vi "I(V)_MFLI_PK_v4.0_measure X_JA.vi"() -> ()   [LabVIEW 2016]
uses:
  <instrlib>/Zurich Instruments LabOne/Public/Data/ziTypeDemodSampleSingle.ctl
  <instrlib>/Zurich Instruments LabOne/Public/Configure/ziSetValueDouble.vi
  <instrlib>/Zurich Instruments LabOne/Public/Configure/ziGetValueDemodSampleEx.vi
  <instrlib>/Zurich Instruments LabOne/Zurich Instruments LabOne.lvlib
panel:
  in  "MFLI Average":i32=100
  out "Resistance (ohm)":dbl=199454.37084208988 format="%#_13g"
  out "R vs V":cluster{dbl, "Field Reading":dbl}[](graph)=[{-1.8658364793807455e-07, "Field Reading"=-5985375.99761147}, {0.0008047217670174316, "Field Reading"=58034.083264977155}, {0.006188920855878626, "Field Reading"=189132.7586129212}, {0.008661983047703013, "Field Reading"=188771.34545897675}, {0.011677225951461827, "Field Reading"=183691.50568817492}, {0.014699115782360871, "Field Reading"=182636.4454009372}, {0.01781292120181203, "Field Reading"=183587.98996634493}, {0.021555256828840116, "Field Reading"=183256.70096481865}, {0.0236969881625879, "Field Reading"=179811.4531572173}, {0.0268382090303007, "Field Reading"=180203.76836486548}, {0.029778473153180697, "Field Reading"=178163.04487238626}, {0.03264072061889641, "Field Reading"=177260.15531158168}, {0.03559268653650901, "Field Reading"=176483.75528751378}, {0.03873600657471659, "Field Reading"=175874.83449727614}, {0.04159271297620211, "Field Reading"=175096.07383776281}, {0.04461900983799323, "Field Reading"=175146.9956324693}, {0.047516661430038264, "Field Reading"=174476.80666701734}, {0.0504431481228055, "Field Reading"=173129.08596330334}, {0.05326559443241551, "Field Reading"=172453.48332366438}, {0.05635116215561627, "Field Reading"=172454.36285971096}, {0.05918470364886106, "Field Reading"=171294.32380982584}, {0.05678849392995935, "Field Reading"=171842.86563527162}, {0.054558516660547965, "Field Reading"=172513.929844976}, {0.051666443518018905, "Field Reading"=173796.56781855557}, {0.04875716378884139, "Field Reading"=174499.4091901828}, {0.0456833897857083, "Field Reading"=174535.45413851336}, {0.042800744827053996, "Field Reading"=175186.85452909407}, {0.039896162946778085, "Field Reading"=176752.27575774945}, {0.03703992879123455, "Field Reading"=177663.86883334795}, {0.033907725820892756, "Field Reading"=178420.7731026628}, {0.03089869564146004, "Field Reading"=179323.20960562778}, {0.02803035775972007, "Field Reading"=180424.85149037742}, {0.025103485234444375, "Field Reading"=181589.56255323917}, {0.022127320037229455, "Field Reading"=182831.19207563458}, {0.018925033481086973, "Field Reading"=183900.02003839472}, {0.016003338204844515, "Field Reading"=185570.844111978}, {0.012833497613697193, "Field Reading"=184726.78806555786}, {0.009242471962369856, "Field Reading"=186663.0219404325}, {0.006920822778265618, "Field Reading"=193194.64843788292}, {0.003691571307431316, "Field Reading"=189516.5384092014}, {0.0006248907026203935, "Field Reading"=245378.58047363066}, {-0.003117354688106838, "Field Reading"=193257.8984573591}, {-0.0056859382105631, "Field Reading"=191750.4865108771}, {-0.009295137492491059, "Field Reading"=188124.6786582557}, {-0.011703624788450663, "Field Reading"=183784.45614350797}, {-0.014684616339435234, "Field Reading"=182594.47367590445}, {-0.017656252480306167, "Field Reading"=181522.4648897164}, {-0.021536320145377395, "Field Reading"=183073.0065008859}, {-0.023776338991157248, "Field Reading"=179902.69628193657}, {-0.02683039873562931, "Field Reading"=179048.69288689917}, {-0.02970635498439313, "Field Reading"=178092.35013403418}, {-0.03282717027461627, "Field Reading"=178316.52407242588}, {-0.0357040978348346, "Field Reading"=176565.27745126106}, {-0.03875578532753679, "Field Reading"=176647.4269850455}, {-0.041619448848785344, "Field Reading"=175105.06273454835}, {-0.04446301220372863, "Field Reading"=174361.80115734783}, {-0.047437563265043454, "Field Reading"=173725.38479738982}, {-0.05034131671911892, "Field Reading"=173073.2288626541}, {-0.053256468366072576, "Field Reading"=172451.00022738258}, {-0.0563362493767472, "Field Reading"=172462.9539218683}, {-0.05922969457985778, "Field Reading"=171306.588457977}, {-0.05679673949763216, "Field Reading"=171860.06155604066}, {-0.05447822001043159, "Field Reading"=172554.1170355251}, {-0.05166621111556194, "Field Reading"=173798.50214140327}, {-0.0487808772219617, "Field Reading"=174510.78073533485}, {-0.045882024149101024, "Field Reading"=175254.28303170486}, {-0.04294834146997125, "Field Reading"=176008.44516569734}, {-0.03981978170709573, "Field Reading"=176698.20822447524}, {-0.036958265007040234, "Field Reading"=177605.44590742036}, {-0.03391635528617712, "Field Reading"=177487.04286739047}, {-0.030987288293818763, "Field Reading"=178290.68533858887}, {-0.02801550701885121, "Field Reading"=180415.79582835655}, {-0.025125758010770417, "Field Reading"=181610.02047115946}, {-0.021960262490715438, "Field Reading"=182617.25984553303}, {-0.01887532342134995, "Field Reading"=182299.20269686673}, {-0.01595695359183023, "Field Reading"=185489.84330936617}, {-0.012842639265367215, "Field Reading"=184711.54499441996}, {-0.0092489906287816, "Field Reading"=186773.20728566393}, {-0.006817686490835859, "Field Reading"=187528.08819678446}, {-0.0037725901319319, "Field Reading"=199454.37084208988}]
  out "Set Voltage(V)":dbl=-0.007071067811865454 format="%#_13g"
  out "Time(s)":dbl=126.699 format="%#_13g"
  out "Demod Sample Out 2":T1={"Timestamps (ticks)"=25761655555070, "X (Vrms)"=-1.8914552315921416e-08, "Y (Vrms)"=2.1781200518488673e-09, "Osc Phase (deg)"=5.451671846346326, "Freq (Hz)"=7.919000069023241, "DIO"=0, "AuxIn0 (V)"=0.0003346765006426722, "AuxIn1 (V)"=0.0020019487710669637, "Trigger"=0}
  out "Demod Sample Out":T1={"Timestamps (ticks)"=25761652544510, "X (Vrms)"=-0.0037725901319319, "Y (Vrms)"=0.00040249016544426157, "Osc Phase (deg)"=2.9379567039979744, "Freq (Hz)"=7.919000069023241, "DIO"=0, "AuxIn0 (V)"=0.0010040295019280165, "AuxIn1 (V)"=0.0006673162570223212, "Trigger"=768}
  in  "MFLI Current source/Voltage reader":string="DEV4382"
  out "Imeas (A)":dbl=-1.8914552315921416e-08
  out "Vmeas (V)":dbl=-0.0037725901319319
  in  "Folder":path=path "D:/Pranava/Data/STS/MA1981"
  in  "wait (ms) [Should be > TC]":u32=1000
  out "V vs I":cluster{dbl, "Field Reading":dbl}[](graph)=[{-1.8658364793807455e-07, "Field Reading"=3.117325428052186e-14}, {0.0008047217670174316, "Field Reading"=1.3866364759190934e-08}, {0.006188920855878626, "Field Reading"=3.2722627752418406e-08}, {0.008661983047703013, "Field Reading"=4.588611172231863e-08}, {0.011677225951461827, "Field Reading"=6.356976555728426e-08}, {0.014699115782360871, "Field Reading"=8.048292743593576e-08}, {0.01781292120181203, "Field Reading"=9.702661489500195e-08}, {0.021555256828840116, "Field Reading"=1.1762329407522326e-07}, {0.0236969881625879, "Field Reading"=1.3178797983390163e-07}, {0.0268382090303007, "Field Reading"=1.4893256269735908e-07}, {0.029778473153180697, "Field Reading"=1.671416941403885e-07}, {0.03264072061889641, "Field Reading"=1.8414020094657876e-07}, {0.03559268653650901, "Field Reading"=2.016768425996157e-07}, {0.03873600657471659, "Field Reading"=2.2024757939611033e-07}, {0.04159271297620211, "Field Reading"=2.3754223646807917e-07}, {0.04461900983799323, "Field Reading"=2.5475178536103656e-07}, {0.047516661430038264, "Field Reading"=2.723379819801613e-07}, {0.0504431481228055, "Field Reading"=2.9136148811816346e-07}, {0.05326559443241551, "Field Reading"=3.0886934497255417e-07}, {0.05635116215561627, "Field Reading"=3.267598524106757e-07}, {0.05918470364886106, "Field Reading"=3.455146810034933e-07}, {0.05678849392995935, "Field Reading"=3.304675682637314e-07}, {0.054558516660547965, "Field Reading"=3.1625571749235085e-07}, {0.051666443518018905, "Field Reading"=2.972811498323656e-07}, {0.04875716378884139, "Field Reading"=2.7941162675056453e-07}, {0.0456833897857083, "Field Reading"=2.6174275026925725e-07}, {0.042800744827053996, "Field Reading"=2.4431481997952013e-07}, {0.039896162946778085, "Field Reading"=2.2571795907996334e-07}, {0.03703992879123455, "Field Reading"=2.0848318250898104e-07}, {0.033907725820892756, "Field Reading"=1.9004359879879207e-07}, {0.03089869564146004, "Field Reading"=1.7230728643220945e-07}, {0.02803035775972007, "Field Reading"=1.553575215840763e-07}, {0.025103485234444375, "Field Reading"=1.382429963566019e-07}, {0.022127320037229455, "Field Reading"=1.2102595725611036e-07}, {0.018925033481086973, "Field Reading"=1.0290936062506028e-07}, {0.016003338204844515, "Field Reading"=8.623842975671172e-08}, {0.012833497613697193, "Field Reading"=6.947285636311016e-08}, {0.009242471962369856, "Field Reading"=4.95142094362926e-08}, {0.006920822778265618, "Field Reading"=3.58230563539178e-08}, {0.003691571307431316, "Field Reading"=1.9478887375309313e-08}, {0.0006248907026203935, "Field Reading"=2.546639162286403e-09}, {-0.003117354688106838, "Field Reading"=-1.613054220805707e-08}, {-0.0056859382105631, "Field Reading"=-2.965279678829166e-08}, {-0.009295137492491059, "Field Reading"=-4.940945312856299e-08}, {-0.011703624788450663, "Field Reading"=-6.368125484623083e-08}, {-0.014684616339435234, "Field Reading"=-8.042201959244206e-08}, {-0.017656252480306167, "Field Reading"=-9.726758884104614e-08}, {-0.021536320145377395, "Field Reading"=-1.176378787730958e-07}, {-0.023776338991157248, "Field Reading"=-1.3216221592307814e-07}, {-0.02683039873562931, "Field Reading"=-1.4984973251146514e-07}, {-0.02970635498439313, "Field Reading"=-1.668030937995698e-07}, {-0.03282717027461627, "Field Reading"=-1.8409494266096748e-07}, {-0.0357040978348346, "Field Reading"=-2.022147182629967e-07}, {-0.03875578532753679, "Field Reading"=-2.193962628780195e-07}, {-0.041619448848785344, "Field Reading"=-2.376827271515194e-07}, {-0.04446301220372863, "Field Reading"=-2.55004318082286e-07}, {-0.047437563265043454, "Field Reading"=-2.7306063141185913e-07}, {-0.05034131671911892, "Field Reading"=-2.908671494137798e-07}, {-0.053256468366072576, "Field Reading"=-3.0882087257164117e-07}, {-0.0563362493767472, "Field Reading"=-3.266571057472985e-07}, {-0.05922969457985778, "Field Reading"=-3.4575257795404255e-07}, {-0.05679673949763216, "Field Reading"=-3.3048248082415414e-07}, {-0.05447822001043159, "Field Reading"=-3.1571672091263823e-07}, {-0.05166621111556194, "Field Reading"=-2.9727650399153655e-07}, {-0.0487808772219617, "Field Reading"=-2.795293048166655e-07}, {-0.045882024149101024, "Field Reading"=-2.6180258396766603e-07}, {-0.04294834146997125, "Field Reading"=-2.4401295875058126e-07}, {-0.03981978170709573, "Field Reading"=-2.2535475660573288e-07}, {-0.036958265007040234, "Field Reading"=-2.0809195809404015e-07}, {-0.03391635528617712, "Field Reading"=-1.9109200727130116e-07}, {-0.030987288293818763, "Field Reading"=-1.738020594568433e-07}, {-0.02801550701885121, "Field Reading"=-1.5528300551634913e-07}, {-0.025125758010770417, "Field Reading"=-1.3835006430584323e-07}, {-0.021960262490715438, "Field Reading"=-1.2025294054510809e-07}, {-0.01887532342134995, "Field Reading"=-1.0354035092921649e-07}, {-0.01595695359183023, "Field Reading"=-8.602602335059763e-08}, {-0.012842639265367215, "Field Reading"=-6.952808101819074e-08}, {-0.0092489906287816, "Field Reading"=-4.9519900435374284e-08}, {-0.006817686490835859, "Field Reading"=-3.63555484215338e-08}, {-0.0037725901319319, "Field Reading"=-1.8914552315921416e-08}]
  out "data":dbl[](array[numeric])=[-0.0037725901319319, -1.8914552315921416e-08, 199454.37084208988, -0.0049999999999999845, 126.699]
  in  "Step":dbl[](array[numeric])=[0.0001, 0.0001, 0.0001] min=-3000.0 max=3000.0 format="%.1e"
  in  "To":dbl[](array[numeric])=[0.003, -0.003, 0.0] min=-3000.0 max=3000.0 format="%.1e"
  in  "From":dbl[](array[numeric])=[0.0, 0.003, -0.003] min=-3000.0 max=3000.0 format="%.1e"
  in  "file name":string="022_MA1981_Dev007_baseT_I(V)_7.919Hz"
  out "File path":path=path "D:/Pranava/Data/STS/MA1981/001_MA1981_Dev007_4K_I(V)_7.919Hz.dat"
  # ".dat"
  # "Set MFLI Voltage output (V)"
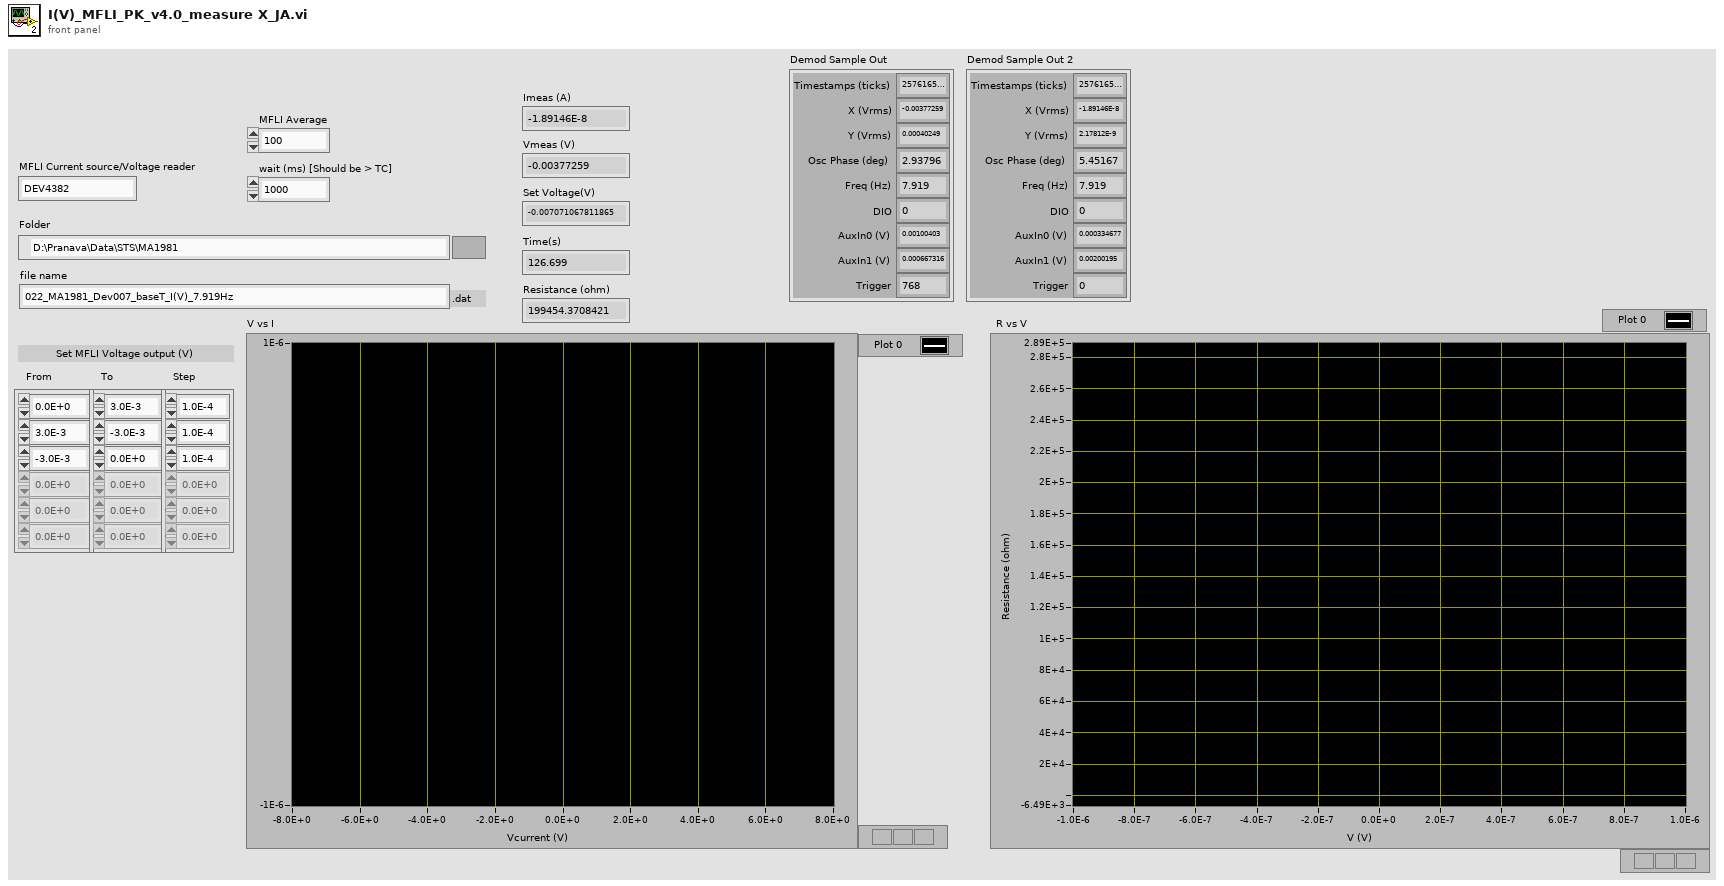
[diagram p1: front panel]
types:
  T1 = typedef "Zurich Instruments LabOne.lvlib/ziTypeDemodSampleSingle.ctl" = cluster{"Timestamps (ticks)":u64, "X (Vrms)":dbl, "Y (Vrms)":dbl, "Osc Phase (deg)":dbl, "Freq (Hz)":dbl, "DIO":u32, "AuxIn0 (V)":dbl, "AuxIn1 (V)":dbl, "Trigger":u32}
  T2 = enum16{"open", "replace", "create", "open or create", "replace or create", "replace or create with confirmation"}
  T3 = typedef "Zurich Instruments LabOne.lvlib/ziTypeHandle.ctl" = cluster{"handleValid":bool, "Conn":u64, "Path Prefix":string, "Handle":u64, "Connected":bool, "Clockbase(s)":dbl}
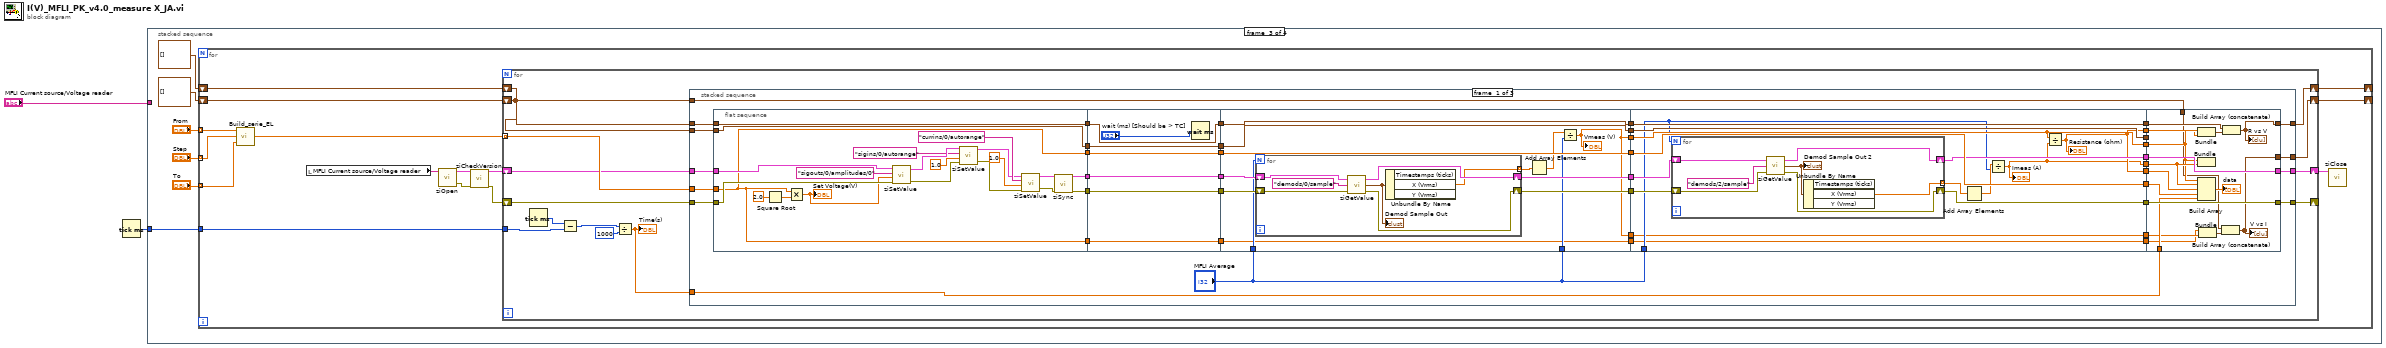
[diagram p0: block diagram]
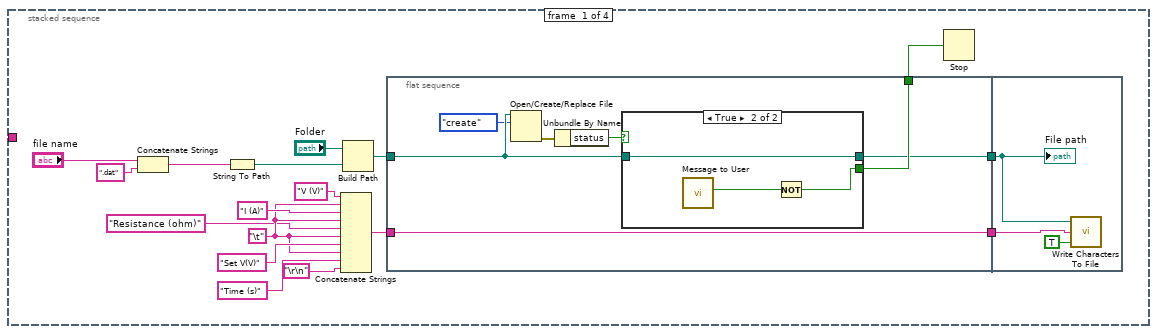
[diagram p2: hidden frame]
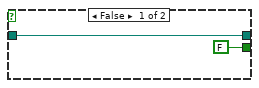
[diagram p3: hidden frame]
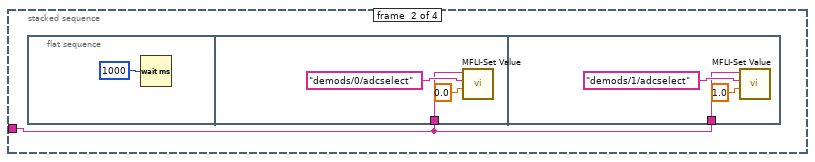
[diagram p4: hidden frame]
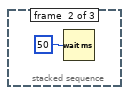
[diagram p5: hidden frame]
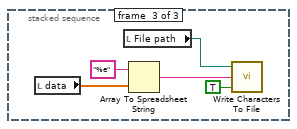
[diagram p6: hidden frame]
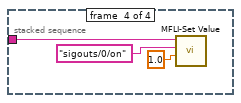
[diagram p7: hidden frame]
diagram:
  n1 = Tick Count (ms)() -> (millisecond timer value=w1:u32)
  n2 = stacked-sequence {
    tunnel: "MFLI Current source/Voltage reader" -> [_ w35 _ w214]
    tunnel: w1 -> [_ _ w44 _]
    frame #0 {
      w4 = "\t"
      n3 = Concatenate Strings("file name", ".dat" ("string")) -> (w16:string)
      n4 = String To Path(string=w16) -> (path=w8:path)
      n5 = Concatenate Strings("V (V)" ("string"), w4, "I (A)" ("string"), w4, "Resistance (ohm)", w4, "Set V(V)" ("string"), w4, "Time (s)", "\r\n") -> (w17:string)
      n6 = Build Path(base path="Folder", name or relative path=w8) -> (appended path=w7:path)
      n7 = flat-sequence {
        tunnel: w7 -> [w23]
        tunnel: w17 -> [w26]
        tunnel: [w26] -> w19
        tunnel: [w25] -> w14
        tunnel: [w24] -> w18
        tunnel: w19 -> [w33]
        tunnel: w18 -> [w32]
        frame #0 {
          n8 = Open/Create/Replace File(file path (use dialog)=w23, operation (0:open)=T2."create") -> (error out=w22:errorcluster)  [unwired: 4 in, 2 out]
          n9 = Unbundle By Name(w22) -> ("status"=w20:bool)
          n10 = case shown="True" w20 {
            tunnel: [FALSE ("Yes") w30] -> w25
            tunnel: [w27 w29] -> w24
            tunnel: w23 -> [w27 w29]
            frame False {
            }
            frame True {
              n11 = call "Message to User"() -> ("Yes"=w31:bool)  [unwired: 10 in, 1 out]
              n12 = Not(x=w31) -> (.not. x?=w30:bool)
            }
          }
        }
        frame #1 {
          n13 = call <vilib>:"Write Characters To File.vi"("append to file? (new file:F)"=TRUE, "character string"=w33, "file path (dialog if empty)"=w32) -> ()  [unwired: 2 in, 1 out]
          "File path" <- w32
        }
      }
      n14 = Stop(stop? (T)=w14) -> ()
    }
    frame #1 {
      n15 = flat-sequence {
        tunnel: w35 -> [w37]
        tunnel: w35 -> [w40]
        frame #0 {
          n16 = Wait (ms)(milliseconds to wait=u32 1000) -> ()  [unwired: 1 out]
        }
        frame #1 {
          n17 = call "MFLI-Set Value.vi"("Value"=0.0, "Path"="demods/0/adcselect", "MFLI Current source/Voltage reader"=w37) -> ()  [unwired: 9 in]
        }
        frame #2 {
          n18 = call "MFLI-Set Value.vi"("Value"=1.0, "Path"="demods/1/adcselect", "MFLI Current source/Voltage reader"=w40) -> ()  [unwired: 9 in]
        }
      }
    }
    frame #2 {
      n19 = for {
        tunnel: "From" -> [w60] mode=indexing
        tunnel: "To" -> [w59] mode=indexing
        tunnel: "Step" -> [w58] mode=indexing
        shift-right: [w62] -> _
        shift-left: cluster{dbl, "Field Reading":dbl}[] [] -> [w63]
        tunnel: w44 -> [w51]
        shift-right: [w50] -> _
        shift-left: cluster{dbl, "Field Reading":dbl}[] [] -> [w49]
        n20 = call "Build_serie_EL.vi"("end value"=w59, "increment"=w58, "start value"=w60) -> ("output array"=w61:dbl[])
        n21 = local read "MFLI Current source/Voltage reader"() -> (w57:string)
        n22 = call <instrlib>:"ziOpen.vi"("Address"=w57) -> ("Error Out"=w56:errorcluster, "HandleOut"=w55:T3)  [unwired: 3 in, 1 out]
        n23 = call <instrlib>:"ziCheckVersion.vi"("Handle In"=w55, "Error In"=w56) -> ("Handle Out"=w54:T3, "Error Out"=w52:errorcluster)  [unwired: 11 in, 1 out]
        n24 = for {
          tunnel: w61 -> [w77] mode=indexing
          shift-right: [w65] -> w62
          shift-left: w63 -> [w64]
          shift-right: [w74] -> w53
          shift-left: w54 -> [w76]
          shift-right: [w73] -> _
          shift-left: w52 -> [w75]
          tunnel: w51 -> [w69]
          shift-right: [w67] -> w50
          shift-left: w49 -> [w66]
          n25 = Tick Count (ms)() -> (millisecond timer value=w70:u32)
          n26 = Subtract(x=w70, y=w69) -> (x-y=w71:u32)
          n27 = Divide(x=w71, y=1000) -> (x/y=w68:dbl)
          "Time(s)" <- w68
          n28 = stacked-sequence {
            tunnel: w77 -> [w119 _ _]
            tunnel: w64 -> [w120 _ _]
            tunnel: w76 -> [w110 _ _]
            tunnel: w75 -> [w109 _ _]
            tunnel: [w99 _ _] -> w74
            tunnel: [w98 _ _] -> w73
            tunnel: w68 -> [w95 _ _]
            tunnel: [w93 _ _] -> w67
            tunnel: w66 -> [w88 _ _]
            tunnel: [w85 _ _] -> w65
            tunnel: w64 -> [w78 _ _]
            frame #0 {
              n29 = flat-sequence {
                tunnel: [w141] -> w116
                tunnel: [w121] -> w115
                tunnel: w119 -> [w121]
                tunnel: w120 -> [w141]
                tunnel: [w124] -> w112
                tunnel: [w125] -> w111
                tunnel: w110 -> [w127]
                tunnel: w109 -> [w126]
                tunnel: w88 -> [w123]
                tunnel: [w123] -> w92
                tunnel: [w121] -> w82
                tunnel: w116 -> [w148]
                tunnel: [w148] -> w118
                tunnel: w115 -> [w147]
                tunnel: [w147] -> w117
                tunnel: [w145] -> w114
                tunnel: [w144] -> w113
                tunnel: w112 -> [w144]
                tunnel: w111 -> [w145]
                tunnel: w92 -> [w143]
                tunnel: [w143] -> w91
                tunnel: w82 -> [w142]
                tunnel: [w142] -> w81
                tunnel: [w150] -> w108
                tunnel: [w161] -> w106
                tunnel: [w160] -> w104
                tunnel: w113 -> [w159]
                tunnel: w114 -> [w158]
                tunnel: w118 -> [w161]
                tunnel: w117 -> [w160]
                tunnel: [w157] -> w102
                tunnel: [w156] -> w101
                tunnel: w91 -> [w155]
                tunnel: [w155] -> w90
                tunnel: "MFLI Average" -> [w152]
                tunnel: "MFLI Average" -> [w151]
                tunnel: [w150] -> w83
                tunnel: w81 -> [w149]
                tunnel: [w149] -> w80
                tunnel: w108 -> [w177]
                tunnel: [w177] -> w107
                tunnel: w106 -> [w183]
                tunnel: [w183] -> w105
                tunnel: w104 -> [w182]
                tunnel: [w182] -> w103
                tunnel: w102 -> [w181]
                tunnel: w101 -> [w180]
                tunnel: [w179] -> w100
                tunnel: [w178] -> w97
                tunnel: [w172] -> w96
                tunnel: [w175] -> w94
                tunnel: w90 -> [w176]
                tunnel: [w176] -> w89
                tunnel: [w175] -> w87
                tunnel: "MFLI Average" -> [w171]
                tunnel: [w170] -> w84
                tunnel: w83 -> [w170]
                tunnel: w80 -> [w169]
                tunnel: [w169] -> w79
                tunnel: w107 -> [w200]
                tunnel: w105 -> [_]
                tunnel: w103 -> [w206]
                tunnel: [w205] -> w99
                tunnel: w100 -> [w205]
                tunnel: [w204] -> w98
                tunnel: w97 -> [w204]
                tunnel: w96 -> [w203]
                tunnel: w95 -> [w202]
                tunnel: w94 -> [w199]
                tunnel: [w198] -> w93
                tunnel: w89 -> [w197]
                tunnel: w87 -> [w196]
                tunnel: [w193] -> w85
                tunnel: w84 -> [w195]
                tunnel: w79 -> [w194]
                tunnel: w78 -> [w191]
                frame #0 {
                  n30 = Square Root(x=2.0) -> (sqrt(x)=w140:dbl)
                  n31 = Multiply(x=w121, y=w140) -> (x*y=w122:dbl)
                  "Set Voltage(V)" <- w122
                  n32 = call-poly <instrlib>:"ziSetValue.vi"("Error In"=w126, "Value"=w122, "Path"="sigouts/0/amplitudes/0", "Handle In"=w127) -> ("Error Out"=w134:errorcluster, "Handle Out"=w137:T3)  [unwired: 1 in]
                  n33 = call-poly <instrlib>:"ziSetValue.vi"("Error In"=w134, "Value"=1.0, "Path"="sigins/0/autorange", "Handle In"=w137) -> ("Error Out"=w130:errorcluster, "Handle Out"=w131:T3)  [unwired: 1 in]
                  n34 = call-poly <instrlib>:"ziSetValue.vi"("Error In"=w130, "Value"=1.0, "Path"="currins/0/autorange", "Handle In"=w131) -> ("Error Out"=w128:errorcluster, "Handle Out"=w129:T3)  [unwired: 1 in]
                  n35 = call <instrlib>:"ziSync.vi"("Handle In"=w129, "Error In"=w128) -> ("Handle Out"=w125:T3, "Error Out"=w124:errorcluster)  [unwired: 12 in]
                }
                frame #1 {
                  n36 = Wait (ms)(milliseconds to wait="wait (ms) [Should be > TC]") -> ()  [unwired: 1 out]
                }
                frame #2 {
                  n37 = for {
                    N: w151 -> [_]
                    tunnel: [w162] -> w154 mode=indexing
                    shift-right: [w163] -> w156
                    shift-left: w159 -> [w166]
                    shift-right: [w164] -> w157
                    shift-left: w158 -> [w165]
                    n38 = call-poly <instrlib>:"ziGetValue.vi"("error in"=w166, "Path"="demods/0/sample", "Handle In"=w165) -> ("error out"=w163:errorcluster, "Demod Sample Out"=w167:T1, "Handle Out"=w164:T3)
                    "Demod Sample Out" <- w167
                    n39 = Unbundle By Name(w167) -> ("X (Vrms)"=w162:dbl)  [unwired: 2 out]
                  }
                  n40 = Add Array Elements(numeric array=w154) -> (sum=w153:dbl)
                  n41 = Divide(x=w153, y=w152) -> (x/y=w150:dbl)
                  "Vmeas (V)" <- w150
                }
                frame #3 {
                  n42 = for {
                    N: w171 -> [_]
                    tunnel: [w184] -> w174 mode=indexing
                    shift-right: [w186] -> w179
                    shift-left: w181 -> [w188]
                    shift-right: [w185] -> w178
                    shift-left: w180 -> [w187]
                    n43 = call-poly <instrlib>:"ziGetValue.vi"("error in"=w187, "Path"="demods/2/sample", "Handle In"=w188) -> ("error out"=w185:errorcluster, "Demod Sample Out"=w189:T1, "Handle Out"=w186:T3)
                    "Demod Sample Out 2" <- w189
                    n44 = Unbundle By Name(w189) -> ("X (Vrms)"=w184:dbl)  [unwired: 2 out]
                  }
                  n45 = Add Array Elements(numeric array=w174) -> (sum=w173:dbl)
                  n46 = Divide(x=w173, y=w171) -> (x/y=w172:dbl)
                  "Imeas (A)" <- w172
                  n47 = Divide(x=w177, y=w172) -> (x/y=w175:dbl)
                  "Resistance (ohm)" <- w175
                }
                frame #4 {
                  n48 = Bundle(w200, w199) -> (w201:cluster{dbl, dbl})  [unwired: 1 in]
                  n49 = Bundle(w200, w203) -> ()  [unwired: 1 in, 1 out]
                  n50 = Build Array(w200, w203, w196, w206, w202) -> (→"data":dbl[])
                  n51 = Bundle(w194, w195) -> (w192:cluster{dbl, dbl})  [unwired: 1 in]
                  n52 = Build Array (concatenate)(w191, w192) -> (w193:cluster{dbl, "Field Reading":dbl}[])
                  "V vs I" <- w193
                  n53 = Build Array (concatenate)(w197, w201) -> (w198:cluster{dbl, "Field Reading":dbl}[])
                  "R vs V" <- w198
                }
              }
            }
            frame #1 {
              n54 = Wait (ms)(milliseconds to wait=u32 50) -> ()  [unwired: 1 out]
            }
            frame #2 {
              n55 = local read "data"() -> (w209:dbl[])
              n56 = local read "File path"() -> (w211:path)
              n57 = Array To Spreadsheet String(array=w209, 3:"%e" ("format string")) -> (spreadsheet string=w212:string)  [unwired: 1 in]
              n58 = call <vilib>:"Write Characters To File.vi"("append to file? (new file:F)"=TRUE, "character string"=w212, "file path (dialog if empty)"=w211) -> ()  [unwired: 2 in, 1 out]
            }
          }
        }
        n59 = call <instrlib>:"ziClose.vi"("Handle In"=w53) -> ()  [unwired: 1 in, 4 out]
      }
    }
    frame #3 {
      n60 = call "MFLI-Set Value.vi"("Value"=1.0, "Path"="sigouts/0/on", "MFLI Current source/Voltage reader"=w214) -> ()  [unwired: 9 in]
    }
  }
